vi "parseCountFromLine.vi"(8 "error in (no error)":errorcluster, 9 "engineeringStatus":string, 10 "line":u32, 11 "DomeCommunicator in":refnum<class "DomeCommunicator.lvclass">) -> (0 "error out":errorcluster, 2 "value":u32, 3 "DomeCommunicator out":refnum<class "DomeCommunicator.lvclass">)   [LabVIEW 2016, in "DomeCommunicator.lvclass"]
uses:
  DomeCommunicator.lvclass
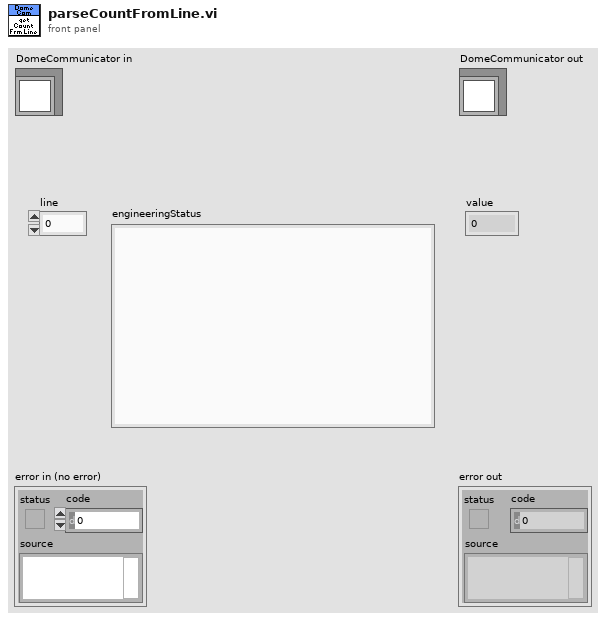
[diagram p1: front panel]
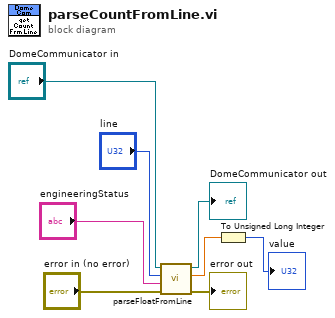
[diagram p0: block diagram]
diagram:
  n1 = call "parseFloatFromLine.vi"("error in (no error)"="error in (no error)", "engineeringStatus"="engineeringStatus", "line"="line", "DomeCommunicator in"="DomeCommunicator in") -> ("error out"=→"error out":errorcluster, "value"=w2:sgl, "DomeCommunicator out"=→"DomeCommunicator out":refnum<class "DomeCommunicator.lvclass">)  [unwired: 5 in]
  n2 = To Unsigned Long Integer(number=w2) -> (unsigned 32bit integer=→"value":u32)
